vi "tracker status to integer.vi"(10 "tracker status":T1) -> (2 "status integer":u32)   [LabVIEW 2010]
uses:
  tracker status.ctl
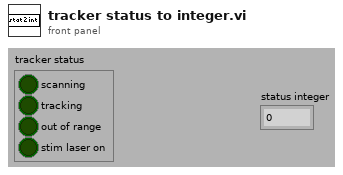
[diagram p1: front panel]
types:
  T1 = typedef "tracker status.ctl" = cluster{"scanning":bool, "tracking":bool, "out of range":bool, "stim laser on":bool}
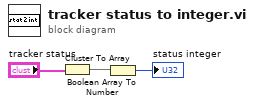
[diagram p0: block diagram]
diagram:
  n1 = Cluster To Array(cluster="tracker status") -> (array=w2:bool[])
  n2 = Boolean Array To Number(Boolean array=w2) -> (number=→"status integer":u32)
